vi "Aktualizacja położenia i orientacji z odczytu GPS.vi"(6 "Azymut robota\n pocz/nowy":dbl caption="Azymut robota pocz/nowy" min=0.0 max=360.0, 9 "Parametry odwzorowania Ziemi (WGS84)":cluster{"a":dbl, "b":dbl}, 10 "Odczyt GPS":bool, 11 "Cluster in":refnum<vi>) -> (1 "Rzeczywista odległość robota od startu [m]":cluster{"X [m]":dbl, "Y [m]":dbl}, 3 "Aktualne położenie":T1)   [LabVIEW 2015, in "Biblioteka moduł map v3.lvlib"]
uses:
  Pomocnicze/Pomocnicze.lvlib
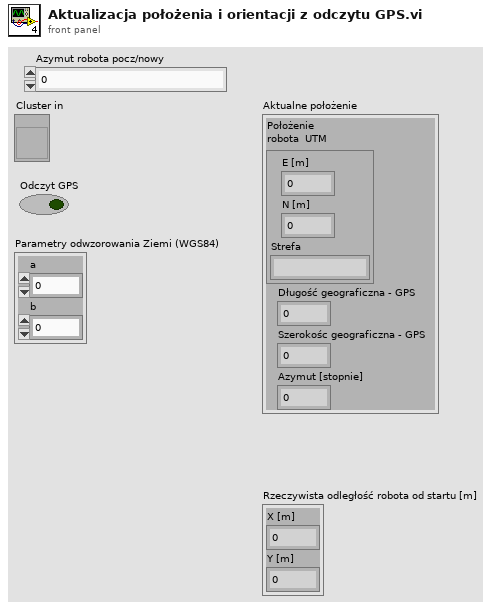
[diagram p1: front panel]
types:
  T1 = cluster{"Położenie \nrobota  UTM":cluster{"E [m]":ext, "N [m]":ext, "Strefa":string}, "Długość geograficzna - GPS":dbl, "Szerokośc geograficzna - GPS":dbl, "Azymut [stopnie]":dbl}
  T2 = cluster{"UTM":cluster{"E [m]":ext, "N [m]":ext, "Strefa":string}, "Piksele":cluster{"X":i32, "Y":i32}}
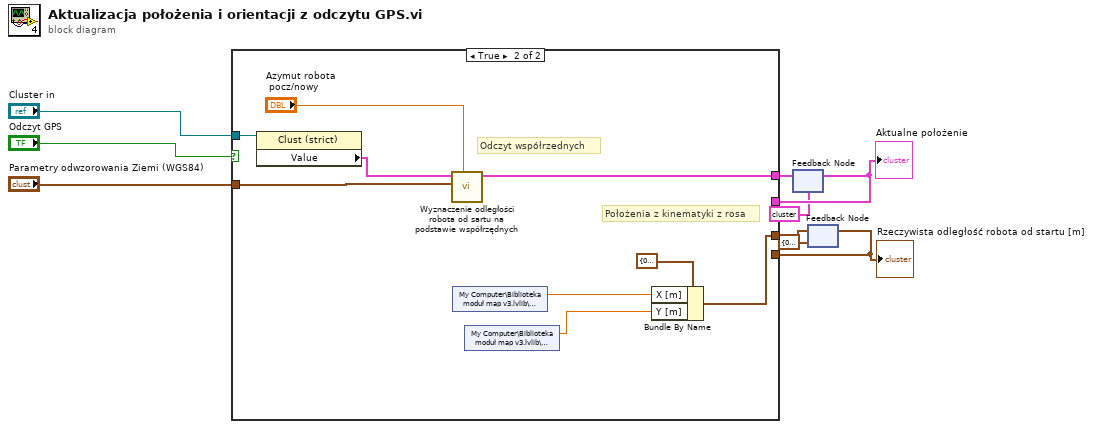
[diagram p0: block diagram]
diagram:
  n1 = feedback #1(T1 {"Położenie \nrobota  UTM"={"E [m]"=0.0, "N [m]"=0.0, "Strefa"=""}, "Długość geograficzna - GPS"=0.0, "Szerokośc geograficzna - GPS"=0.0, "Azymut [stopnie]"=0.0} ("Aktualne położenie")) -> (w5:T1)
  "Aktualne położenie" <- w5
  n2 = feedback #2(cluster{"X [m]":dbl, "Y [m]":dbl} {"X [m]"=0.0, "Y [m]"=0.0} ("Rzeczywista odległość robota od startu [m]")) -> (w3:cluster{"X [m]":dbl, "Y [m]":dbl})
  "Rzeczywista odległość robota od startu [m]" <- w3
  n3 = case shown="True" "Odczyt GPS" {
    tunnel: "Parametry odwzorowania Ziemi (WGS84)" -> [_ w20]
    tunnel: "Cluster in" -> [_ w18]
    tunnel: [w11 w16] -> w6
    tunnel: [w10 w14] -> w4
    tunnel: w5 -> [w11 _]
    tunnel: w3 -> [w10 _]
    frame False {
    }
    frame True {
      # "Położenia z kinematyki z rosa"
      # "Odczyt współrzednych"
      n4 = property class="Clust (strict)"(reference=w18) -> ("Value"=w19:T2)  [unwired: 1 in, 2 out]
      n5 = call "Wyznaczenie odległości robota od sartu na podstawie współrzędnych.vi"("Azymut robota\n pocz/nowy"="Azymut robota\n pocz/nowy", "Parametry odwzorowania Ziemi (WGS84)"=w20, "Pocz. poł."=w19) -> ("Aktualne położenie"=w16:T1)  [unwired: 6 in, 2 out]
      n6 = shared-variable "My Computer\\Biblioteka moduł map v3.lvlib\\Zmienne współdzielone moduł offline.lvlib\\Pozycja X"() -> (w13:dbl)  [unwired: 1 in, 1 out]
      n7 = shared-variable "My Computer\\Biblioteka moduł map v3.lvlib\\Zmienne współdzielone moduł offline.lvlib\\Pozycja Y"() -> (w12:dbl)  [unwired: 1 in, 1 out]
      n8 = Bundle By Name(cluster=cluster{"X [m]":dbl, "Y [m]":dbl} {"X [m]"=0.0, "Y [m]"=0.0} ("Rzeczywista odległość robota od startu [m]"), "X [m]"=w13, "Y [m]"=w12) -> (w14:cluster{"X [m]":dbl, "Y [m]":dbl})
    }
  }
  n9 = feedback-in #1(w6) -> ()
  n10 = feedback-in #2(w4) -> ()
